vi "自动测试类型1统计结果.vi"   [LabVIEW 2010]
uses:
  全局量/自动测试结果.vi
  全局量/试验配置信息.vi
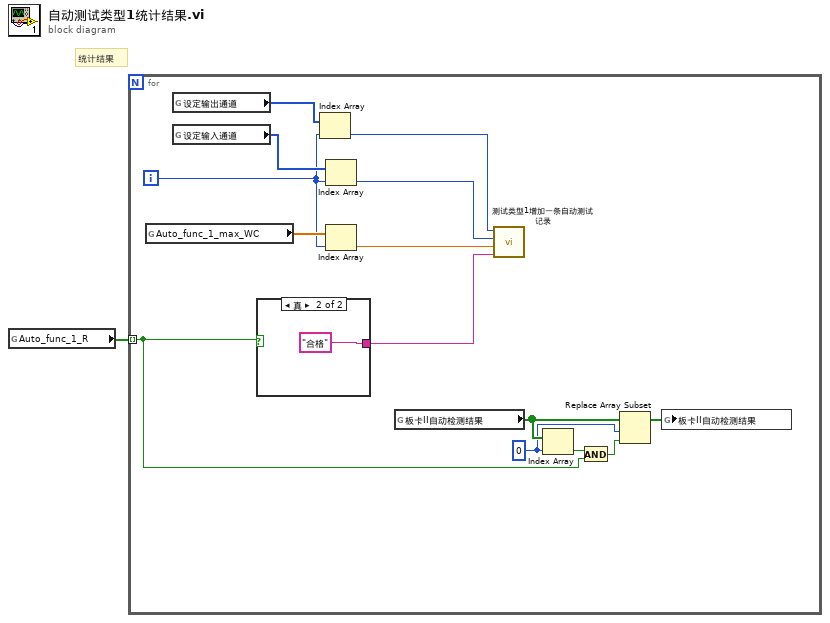
[diagram p0: block diagram]
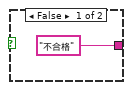
[diagram p2: hidden frame]
diagram:
  # "统计结果"
  n1 = global read "自动测试结果.vi" "Auto_func_1_R"() -> (w1:bool[])
  n2 = for {
    tunnel: w1 -> [w3] mode=indexing
    i -> [w12]
    w5 = 0 ("索引")
    n3 = global read "自动测试结果.vi" "Auto_func_1_max_WC"() -> (w15:dbl[])
    n4 = global read "试验配置信息.vi" "设定输出通道"() -> (w14:i32[])
    n5 = global read "试验配置信息.vi" "设定输入通道"() -> (w13:i32[])
    n6 = case shown="真" w3 {
      tunnel: ["不合格" "合格"] -> w8
      frame False {
      }
      frame True {
      }
    }
    n7 = Index Array(array=w14, index=w12) -> (element=w11:i32)
    n8 = Index Array(array=w13, index=w12) -> (element=w10:i32)
    n9 = Index Array(array=w15, index=w12) -> (element=w9:dbl)
    n10 = global read "试验配置信息.vi" "板卡II自动检测结果"() -> (w6:bool[])
    n11 = call "测试类型1增加一条自动测试记录.vi"("测试结果"=w8, "最大误差"=w9, "输入通道"=w10, "输出通道"=w11) -> ()  [unwired: 8 in]
    n12 = Index Array(array=w6, index=w5) -> (element=w4:bool)
    n13 = And(x=w4, y=w3) -> (x .and. y?=w2:bool)
    n14 = Replace Array Subset(array=w6, new element=w2, index=w5) -> (w7:bool[])
    n15 = global write "试验配置信息.vi" "板卡II自动检测结果"(w7) -> ()
  }
